vi "6733_suspend.vi"(0 "error in":errorcluster) -> (1 "task ID out":u32 format="%x", 3 "error out":errorcluster)   [LabVIEW 2013]
panel:
  out "6733 Status":string="PCI-6733 OK"
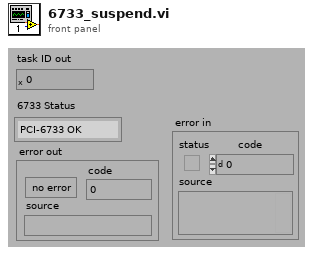
[diagram p1: front panel]
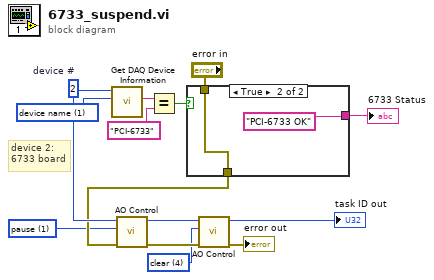
[diagram p0: block diagram]
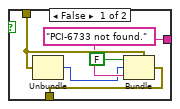
[diagram p2: hidden frame]
diagram:
  w1 = u16 4 items=["start", "pause", "pause at EOC", "resume", "clear", "switch to next buffer", "switch to next buffer at EOC", "new staging list"] ("control code (0: start)")
  w6 = u16 1 items=["start", "pause", "pause at EOC", "resume", "clear", "switch to next buffer", "switch to next buffer at EOC", "new staging list"] ("control code (0: start)")
  w14 = u32 1 items=["NI-DAQ version", "device name", "base address", "data transfer mode for analog input", "data transfer mode for analog output group 1", "data transfer mode for analog output group 2", "data transfer mode for GPCTR 0", "data transfer mode for GPCTR 1", "data transfer mode for digital I/O group 1", "data transfer mode for digital I/O group 2", "device type code", "DMA A level", "DMA B level", "DMA C level", "interrupt A level", "interrupt B level", "reserved", "lpt device mode", "DAQCard-700 counter 1 source", "interrupt generation mode", "device state during suspend mode", "computer name", "serial number", "counter type"] ("information type")
  w8 = u32 2  # device #
  # "device 2:\n6733 board"
  n1 = call "Get DAQ Device Information.vi"("information type"=w14, "task ID or device"=w8) -> ("information string"=w13:string)  [unwired: 7 in, 2 out]
  n2 = Equal?(x=w13, y="PCI-6733") -> (x = y?=w11:bool)
  n3 = case shown="True" w11 {
    tunnel: [w18 "PCI-6733 OK"] -> w10
    tunnel: "error in" -> [w19 w20]
    tunnel: [w17 w20] -> w7
    frame False {
      w18 = "PCI-6733 not found."
      n4 = Unbundle(w19) -> ("code"=w15:i32)  [unwired: 2 out]
      n5 = Bundle(cluster=w19, "status"=FALSE, "code"=w15, "source"=w18) -> (w17:errorcluster)
    }
    frame True {
    }
  }
  "6733 Status" <- w10
  n6 = call "AO Control.vi"("error in (no error)"=w7, "control code (0: start)"=w6, "task ID"=w8) -> ("error out"=w4:errorcluster, "task ID out"=w5:u32)  [unwired: 7 in]
  n7 = call "AO Control.vi"("error in (no error)"=w4, "control code (0: start)"=w1, "task ID"=w5) -> ("error out"=→"error out":errorcluster, "task ID out"=→"task ID out":u32)  [unwired: 7 in]
